vi "SAOMM-connect.vi"(0 "IP":string, 7 "Port":u16, 11 "Signature":u32=9518, 13 "Command.ini":path=path "C:/BonOMM/BonOMM 7.1/BonOMM 7.1.vi" caption="Répertoire de configuration") -> (4 "connection ID":refnum<k5>, 6 "Connexion":bool, 8 "Lecture":bool, 10 "Écriture":bool, 15 "Error OUT":errorcluster)   [LabVIEW 2019]
panel:
  out "SignatureReturned":u32
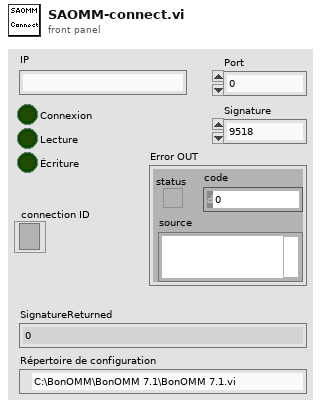
[diagram p1: front panel]
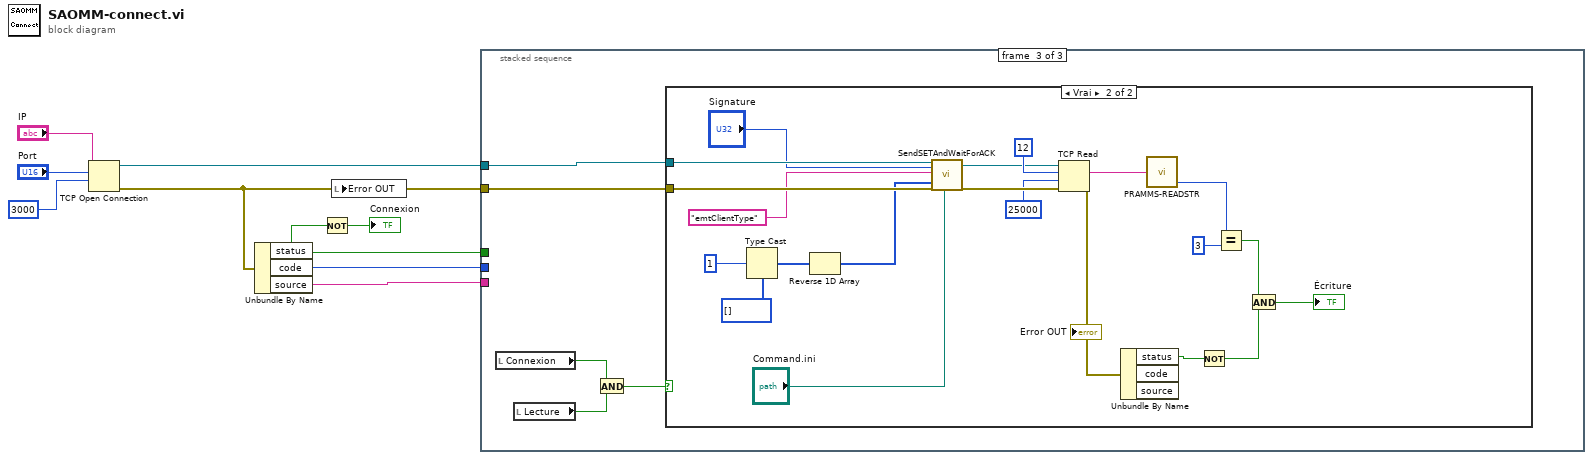
[diagram p0: block diagram]
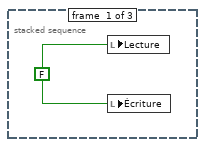
[diagram p2: hidden frame]
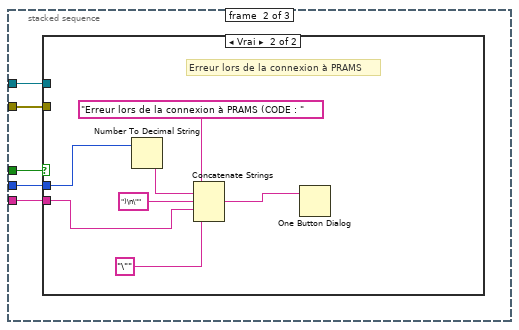
[diagram p3: hidden frame]
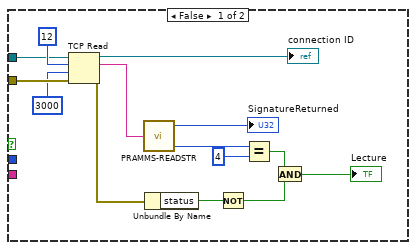
[diagram p4: hidden frame]
diagram:
  n1 = TCP Open Connection(address="IP", remote port or service name="Port", timeout ms (60000)=3000) -> (connection ID=w9:refnum<k5>, error out=w1:errorcluster)  [unwired: 2 in]
  n2 = Unbundle By Name(w1) -> ("status"=w4:bool, "code"=w7:i32, "source"=w6:string)
  n3 = Not(x=w4) -> (.not. x?=→"Connexion":bool)
  n4 = local write "Error OUT"(w1) -> ()
  n5 = stacked-sequence {
    tunnel: w9 -> [_ w15 w37]
    tunnel: w1 -> [_ w14 w38]
    tunnel: w7 -> [_ w13 _]
    tunnel: w6 -> [_ w12 _]
    tunnel: w4 -> [_ w11 _]
    frame #0 {
      w10 = FALSE
      n6 = local write "Lecture"(w10) -> ()
      n7 = local write "Écriture"(w10) -> ()
    }
    frame #1 {
      n8 = case shown="Vrai" w11 {
        tunnel: w15 -> [w28 _]
        tunnel: w14 -> [w27 _]
        tunnel: w13 -> [_ w36]
        tunnel: w12 -> [_ w31]
        frame False {
          n9 = TCP Read(connection ID=w28, bytes to read=12, error in (no error)=w27, 9:3000 ("timeout ms (25000)")) -> (connection ID out=→"connection ID":refnum<k5>, data out=w26:string, error out=w19:errorcluster)  [unwired: 1 in]
          n10 = call "PRAMMS-READSTR.vi"("String"=w26) -> ("Signature"=→"SignatureReturned":u32, "Type"=w25:u32)  [unwired: 1 out]
          n11 = Unbundle By Name(w19) -> ("status"=w23:bool)
          n12 = Not(x=w23) -> (.not. x?=w22:bool)
          n13 = Equal?(x=w25, y=u32 4) -> (x = y?=w21:bool)
          n14 = And(x=w21, y=w22) -> (x .and. y?=→"Lecture":bool)
        }
        frame True {
          # "Erreur lors de la connexion à PRAMS"
          n15 = Number To Decimal String(number=w36) -> (decimal integer string=w35:string)  [unwired: 1 in]
          n16 = Concatenate Strings("Erreur lors de la connexion à PRAMS (CODE : ", w35, ")\n\"", w31, "\"") -> (w32:string)
          n17 = One Button Dialog(message=w32) -> ()  [unwired: 1 in, 1 out]
        }
      }
    }
    frame #2 {
      n18 = local read "Connexion"() -> (w41:bool)
      n19 = local read "Lecture"() -> (w40:bool)
      n20 = And(x=w41, y=w40) -> (x .and. y?=w39:bool)
      n21 = case shown="Vrai" w39 {
        tunnel: w38 -> [_ w61]
        tunnel: w37 -> [_ w62]
        frame False {
        }
        frame True {
          n22 = Type Cast(type=u8[] [], x=u32 1) -> (*(type *) &x=w57:u8[])
          n23 = Reverse 1D Array(array=w57) -> (reversed array=w56:u8[])
          n24 = call "SendSETAndWaitForACK.vi"("connection ID"=w62, "Signature"="Signature", "Active SET"="emtClientType", "Value (little endianed byte array)"=w56, "Error IN"=w61, "path_config"="Command.ini") -> ("connection ID (dup)"=w51:refnum<k5>, "Error OUT"=w50:errorcluster)  [unwired: 12 in]
          n25 = TCP Read(connection ID=w51, bytes to read=12, error in (no error)=w50, 9:25000 ("timeout ms (25000)")) -> (data out=w52:string, error out=w49:errorcluster)  [unwired: 1 in, 1 out]
          "Error OUT" <- w49
          n26 = Unbundle By Name(w49) -> ("status"=w54:bool)  [unwired: 2 out]
          n27 = call "PRAMMS-READSTR.vi"("String"=w52) -> ("Type"=w48:u32)  [unwired: 2 out]
          n28 = Not(x=w54) -> (.not. x?=w45:bool)
          n29 = Equal?(x=w48, y=u32 3) -> (x = y?=w46:bool)
          n30 = And(x=w46, y=w45) -> (x .and. y?=→"Écriture":bool)
        }
      }
    }
  }
